vi "Get Wait Value from Channel.vi"(8 "error in (no error)":errorcluster, 9 "Wait Value Lookup":variant, 10 "Wait Values":dbl[](array[numeric]), 11 "Response":T1) -> (0 "error out":errorcluster, 3 "Response out":T1)   [LabVIEW 2013, in "Instrument Addon Engine.lvlib"]
uses:
  Instrument Addon Engine.lvlib
  Shared/Types/Response RT Configuration Cluster.ctl
  Shared/Types/Response Parameters.ctl
  Shared/Types/Linked Channel Cluster.ctl
  Shared/Types/Response Wait Type.ctl
  Shared/Instrument Addon Shared.lvlib
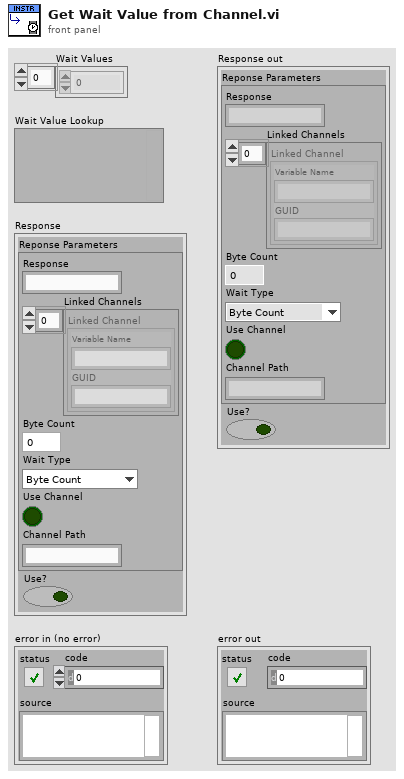
[diagram p1: front panel]
types:
  T1 = typedef "Instrument Addon Shared.lvlib/Response RT Configuration Cluster.ctl" = cluster{"Reponse Parameters":T2, "Use?":bool}
  T2 = typedef "Instrument Addon Shared.lvlib/Response Parameters.ctl" = cluster{"Response":string, "Linked Channels":T3[], "Type Value":dbl, "Wait Type":T4, "Use Channel":bool, "Channel Path":string}
  T3 = typedef "Instrument Addon Shared.lvlib/Linked Channel Cluster.ctl" = cluster{"Variable Name":string, "GUID":string}
  T4 = typedef "Instrument Addon Shared.lvlib/Response Wait Type.ctl" = enum16{"Byte Count", "Wait sec"}
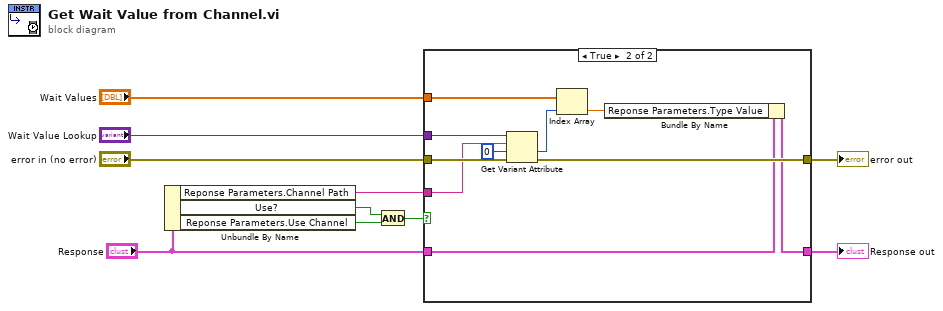
[diagram p0: block diagram]
diagram:
  n1 = Unbundle By Name("Response") -> ("Reponse Parameters.Channel Path"=w4:string, "Use?"=w5:bool, "Reponse Parameters.Use Channel"=w6:bool)
  n2 = And(x=w5, y=w6) -> (x .and. y?=w3:bool)
  n3 = case shown="True" w3 {
    tunnel: "Wait Value Lookup" -> [_ w22]
    tunnel: [w12 w21] -> w9
    tunnel: "error in (no error)" -> [w12 w20]
    tunnel: "Wait Values" -> [_ w19]
    tunnel: w4 -> [_ w18]
    tunnel: "Response" -> [w11 w15]
    tunnel: [w11 w13] -> w1
    frame False {
    }
    frame True {
      n4 = Get Variant Attribute(Variant=w22, name=w18, default value (empty Variant)=0, error in=w20) -> (value=w16:i32, error out=w21:errorcluster)  [unwired: 2 out]
      n5 = Index Array(array=w19, index=w16) -> (element=w14:dbl)
      n6 = Bundle By Name(cluster=w15, "Reponse Parameters.Type Value"=w14) -> (w13:T1)
    }
  }
  "error out" <- w9
  "Response out" <- w1
